vi "GCM_About.vi"(8 "error in":errorcluster, 10 "VI reference":refnum<vi>) -> (0 "error out":errorcluster)   [LabVIEW 2014]
doc: "About window."
uses:
  <vilib>/Platform/browser.llb/Open URL in Default Browser (string).vi
panel:
  out "Info":string="Special thanks for May, TMa and Hooovahh for testing earlier versions of GCM."
  in  "WebPage":bool
  in  "Veritech":bool
  in  "OK Button":bool
  # "VERITECH Sp. z o.o.\nul. Czarnolesna 18\n41-709 Ruda Slaska\nPoland\n(+48) 32 494 49 44"
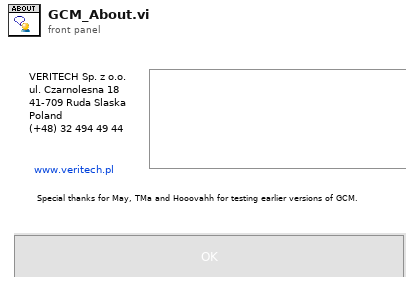
[diagram p1: front panel]
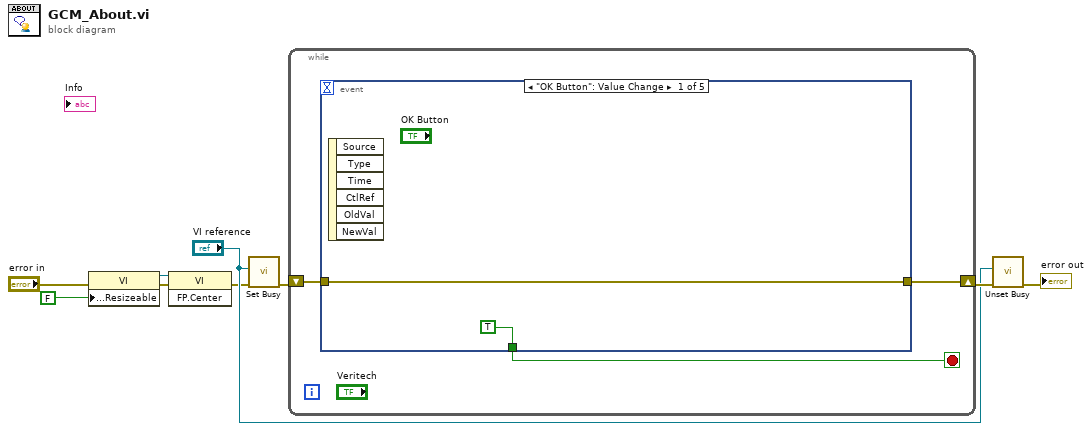
[diagram p0: block diagram]
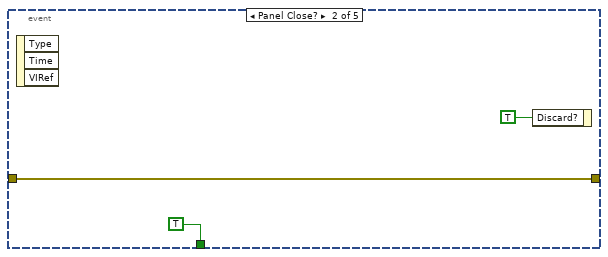
[diagram p2: hidden frame]
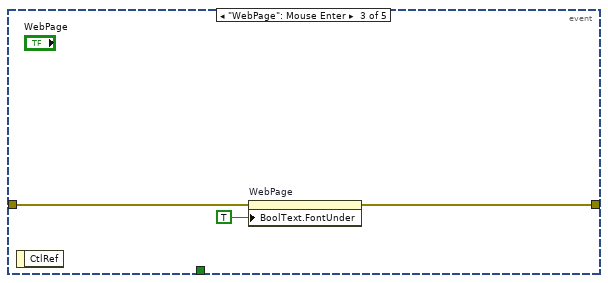
[diagram p3: hidden frame]
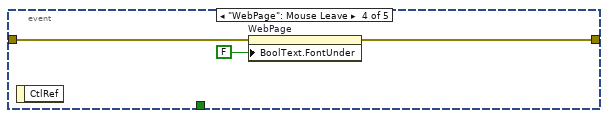
[diagram p4: hidden frame]
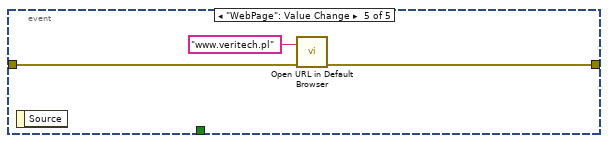
[diagram p5: hidden frame]
diagram:
  n1 = property class="VI"(error in="error in", "Front Panel.Resizeable"=FALSE ("Front Panel Window:Resizable")) -> (reference out=w3:refnum<vi>, error out=w4:errorcluster)  [unwired: 1 in]
  n2 = invoke class="VI" method="FP.Center"(reference=w3, error in=w4) -> (error out=w2:errorcluster)  [unwired: 1 in, 2 out]
  n3 = call <vilib>:"Set Busy.vi"("error in (no error)"=w2, "VI reference (current VI)"="VI reference") -> ("error out"=w1:errorcluster)  [unwired: 8 in, 1 out]
  n4 = while {
    shift-right: [w10] -> w9
    shift-left: w1 -> [w11]
    stop <- w12 stop-if-true
    n5 = event shown="[0] \"OK Button\": Value Change" {
      selector: _ -> [_ _ _ _ _]
      dyn-events: _ -> [_ _ _ _ _]
      timeout: _ -> [_ _ _ _ _]
      tunnel: [TRUE TRUE _ _ _] -> w12
      tunnel: [w13 w16 w19 w21 w24] -> w10
      tunnel: w11 -> [w13 w16 w18 w22 w25]
      event "OK Button": Value Change {
        n6 = event-data() -> ()  [unwired: 7 out]
      }
      event Panel Close? {
        n7 = event-data() -> ()  [unwired: 4 out]
        n8 = event-data("Discard?"=TRUE) -> ()  [unwired: 1 in, 1 out]
      }
      event "WebPage": Mouse Enter {
        n9 = event-data() -> ()  [unwired: 2 out]
        n10 = property on="WebPage" class="Bool"(error in=w18, "BoolText.FontUnder"=TRUE ("Boolean Text.Font:Underline")) -> (error out=w19:errorcluster)  [unwired: 1 in, 1 out]
      }
      event "WebPage": Mouse Leave {
        n11 = event-data() -> ()  [unwired: 2 out]
        n12 = property on="WebPage" class="Bool"(error in=w22, "BoolText.FontUnder"=FALSE ("Boolean Text.Font:Underline")) -> (error out=w21:errorcluster)  [unwired: 1 in, 1 out]
      }
      event "WebPage": Value Change {
        n13 = event-data() -> ()  [unwired: 2 out]
        n14 = call-poly <vilib>:"Open URL in Default Browser.vi"("error in (no error)"=w25, "URL"="www.veritech.pl") -> ("error out"=w24:errorcluster)  [unwired: 5 out]
      }
    }
  }
  n15 = call <vilib>:"Unset Busy.vi"("error in (no error)"=w9, "VI reference (current VI)"="VI reference") -> ("error out"=→"error out":errorcluster)  [unwired: 9 in]
